vi "State_Machine.vi"(8 "error in (no error)":errorcluster caption="entrée d'erreur (pas d'erreur)", 11 "Test_With_Inst en entrée":refnum<class "Test_With_Inst.lvclass">) -> (0 "error out":errorcluster caption="sortie d'erreur", 2 "Json_String":string, 3 "Test_With_Inst en sortie":refnum<class "Test_With_Inst.lvclass">)   [LabVIEW 2020, in "Library Test.lvlib" / "Test_With_Inst.lvclass"]
uses:
  Test_With_Inst.lvclass
  Test (Default)/Test (Default).lvclass
  Test_With_Inst.lvclass/Test_With_Inst.ctl
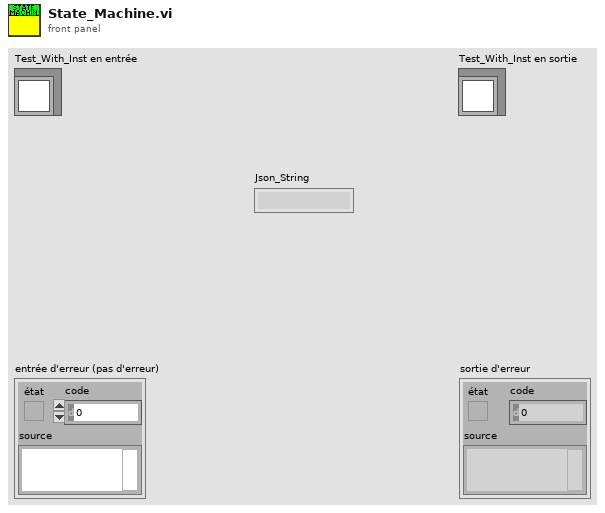
[diagram p1: front panel]
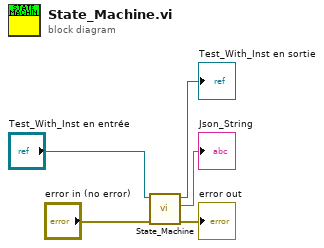
[diagram p0: block diagram]
diagram:
  n1 = call-parent "State_Machine.vi"("error in (no error)"="error in (no error)", "Test (Default) en entrée"="Test_With_Inst en entrée") -> ("error out"=→"error out":errorcluster, "Json_String"=→"Json_String":string, "Test (Default) en sortie"=→"Test_With_Inst en sortie":refnum<class "Test_With_Inst.lvclass">)  [unwired: 7 in]
